vi "ZCAN_Getcn.vi"(8 "error in (no error)":errorcluster caption="错误输入（无错误）", 10 "channelIdx":u32, 11 "device_handle":u32) -> (0 "error out":errorcluster caption="错误输出", 1 "SN out":string)   [LabVIEW 2020, in "zlgcan.lvlib"]
uses:
  zlgcan.lvlib
  bin/zlgcan_wrap.dll
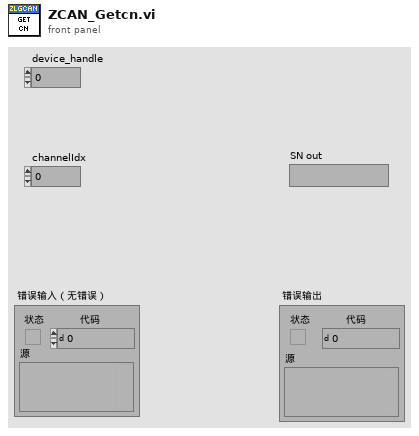
[diagram p1: front panel]
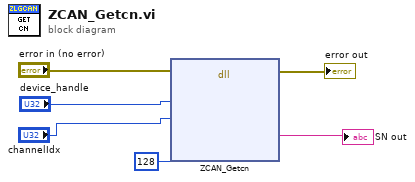
[diagram p0: block diagram]
diagram:
  n1 = dll-call lib="D:/Git/ZLG_USBCANFD/bin/zlgcan_wrap.dll" fn="ZCAN_Getcn" ("ZCAN_StartCAN")(error in="error in (no error)", "device_handle"="device_handle", "channelIdx"="channelIdx", "len"=128) -> (error out=→"error out":errorcluster, "get_sn"=→"SN out":string)  [unwired: 7 in, 1 out]
